vi "testLED.vi"() -> ()   [LabVIEW 2019]
uses:
  <userlib>/KNR OS 4.2 LabVIEW Toolkit/Type Definition/Resource.ctl
  <userlib>/KNR OS 4.2 LabVIEW Toolkit/Type Definition/RC Servo Port.ctl
panel:
  in  "Numeric Control":i32
  in  "Stop Button":bool
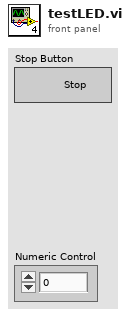
[diagram p1: front panel]
types:
  T1 = typedef "RC Servo Port.ctl" = u16
  T2 = typedef "Resource.ctl" = enum16{"KNRm_DDRC", "KNRm_DDDD", "KNRm_DDDR", "KNRm_DDDC", "KNR", "KNRm_neww"}
  T3 = typedef "KNR3 Reference.ctl" = cluster{"FPGA Session":refnum<class "FPGA Interface Base.lvclass">, "Resource":T2}
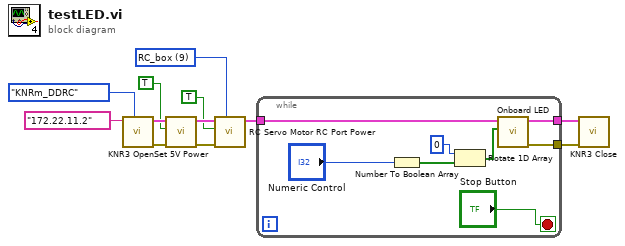
[diagram p0: block diagram]
diagram:
  w5 = T1 9 items=["RC_onboard"=3, "RC_box"=9] ("Port (RC_onboard)")
  n1 = call <userlib>:"KNR3 Open.vi"("Resource"=Resource."KNRm_DDRC", "IP"="172.22.11.2") -> ("error out"=w7:errorcluster, "KNR out"=w11:T3)  [unwired: 8 in]
  n2 = call <userlib>:"Set 5V Power.vi"("error in (no error)"=w7, "5V Power(T)"=TRUE, "KNR in"=w11) -> ("error out"=w9:errorcluster, "KNR out"=w12:T3)  [unwired: 7 in]
  n3 = call <userlib>:"RC Servo Motor RC Port Power.vi"("Port (RC_onboard)"=w5, "error in (no error)"=w9, "RC Power(F)"=TRUE, "KNR in"=w12) -> ("KNR out"=w3:T3)  [unwired: 6 in, 1 out]
  n4 = while {
    tunnel: w3 -> [w20]
    tunnel: [w18] -> w2
    tunnel: [w17] -> w1
    stop <- "Stop Button" stop-if-true
    n5 = Number To Boolean Array(number="Numeric Control") -> (Boolean array=w15:bool[])
    n6 = Rotate 1D Array(1:w15, 2:0 ("n")) -> (0:w14:bool[])
    n7 = call <userlib>:"Onboard LED.vi"("LED List"=w14, "KNR in"=w20) -> ("error out"=w18:errorcluster, "KNR out"=w17:T3)  [unwired: 8 in]
  }
  n8 = call <userlib>:"KNR3 Close.vi"("error in (no error)"=w2, "KNR in"=w1) -> ()  [unwired: 9 in, 1 out]
